vi "ROI entry-User ROI event-Analyse.vi"(8 "error in (no error)":errorcluster, 11 "Event Type":u32) -> (0 "error out":errorcluster, 2 "output cluster":T2 {"ROIs Info []"."Zoom" min=1.0 max=10.0 step=0.10000000149011612; "Last Image Display Event info"."Tool" items=["None", "Selection Tool", "Point Tool", "Line Tool", "Rectangle Tool", "Oval Tool", "Polygon Tool", "ClosedFreehandTool", "Annulus Tool", "Rotated Rectangle Tool", "Zoom Tool", "Pan Tool", "Polyline Tool", "Freehand Tool"]; "Last Image Display Event info"."Type" items=["No Event"=0, "Click Event"=1, "Draw Event"=2, "Size Event"=4, "Scroll Event"=5, "Double Click Event"=8]})   [LabVIEW 2013]
uses:
  Typedefs/ROI Entry screen VI interface 1.ctl
  Typedefs/Last Image Display Event info.ctl
  Typedefs/ROI spec.ctl
  Typedefs/ROI ID Enum.ctl
  Typedefs/ROI info cluster.ctl
  ROI Entry screen/Globals/gl_ROI Entry UI globals.vi
panel:
  out "ROI info cluster (native format)":T1
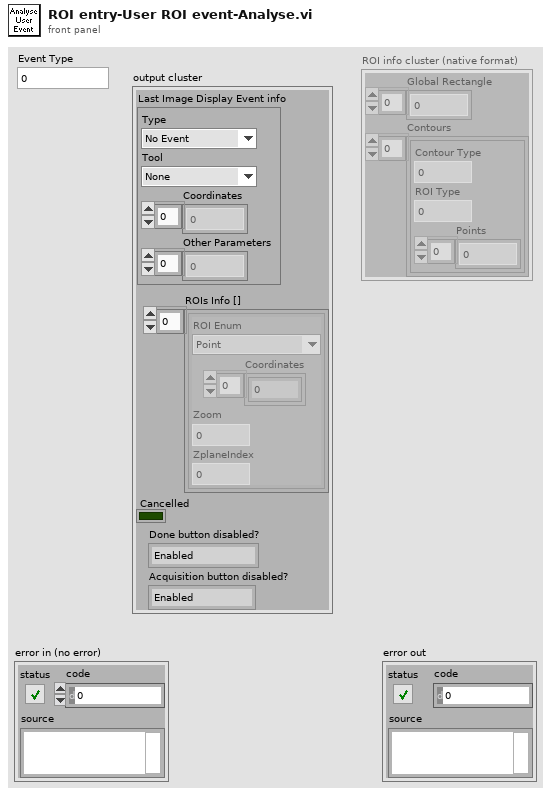
[diagram p1: front panel]
types:
  T1 = typedef "ROI info cluster.ctl" = cluster{"Global Rectangle":i32[], "Contours":cluster{"Contour Type":u32, "ROI Type":u32, "Points":i32[]}[]}
  T2 = typedef "ROI Entry screen VI interface 1.ctl" = cluster{"Last Image Display Event info":T3, "ROIs Info []":T4[], "Cancelled":bool, "Done button disabled?":enum8{"Enabled", "Disabled", "Disabled and Grayed Out"}, "Acquisition button disabled?":enum8{"Enabled", "Disabled", "Disabled and Grayed Out"}}
  T3 = typedef "Last Image Display Event info.ctl" = cluster{"Type":i32, "Tool":i32, "Coordinates":i32[], "Other Parameters":sgl[]}
  T4 = typedef "ROI spec.ctl" = cluster{"Coordinates":i32[], "Zoom":dbl, "ROI Enum":T5, "ZplaneIndex":i32}
  T5 = typedef "ROI ID Enum.ctl" = enum16{"Point", "MiniScan", "Comp. MiniScan", "Rectangle", "Comp. volume", "Arb. plane point"}
  T6 = typedef "ROI entry screen ctrl refs cluster.ctl" = cluster{"Done button":refnum<vi>, "Imaging button":refnum<vi>, "Acquisition button":refnum<vi>, "POI dwell time (us)":refnum<vi>, "Scan dwell time per pixel (us)":refnum<vi>, "# of planes":refnum<vi>, "Zoom":refnum<vi>, "Equal size":refnum<vi>, "Channel":refnum<vi>, "Image Display":refnum<vi>, "Z-Plane Selector":refnum<vi>, "Number of lines left":refnum<vi>, "Z-stack folder path":refnum<vi>, "POI Density":refnum<vi>, "Arb Plane Entry":refnum<vi>, "Whole plane":refnum<vi>, "Clear Last":refnum<vi>, "Clear All":refnum<vi>, "Trial Length (sec)":refnum<vi>, "Palette Type":refnum<vi>, "Intensity slider":refnum<vi>, "# POI":refnum<vi>, "Max Z Proj":refnum<vi>, "Zplane ind":refnum<vi>, "Wavelength (nm)":refnum<vi>, "Number of Trials":refnum<vi>, "Funct stim.trig.enable":refnum<vi>, "Funct stim.trig.delay (s)":refnum<vi>, "Line Mode":refnum<vi>, "Step size (µm)":refnum<vi>, "ROI move mode":refnum<vi>, "Cool-down time (s)":refnum<vi>, "Enable cool-down time":refnum<vi>, "Motor Z ind. (um)":refnum<vi>, "AOL Z ind. (um)":refnum<vi>}
  T7 = enum8{"Enabled", "Disabled", "Disabled and Grayed Out"}
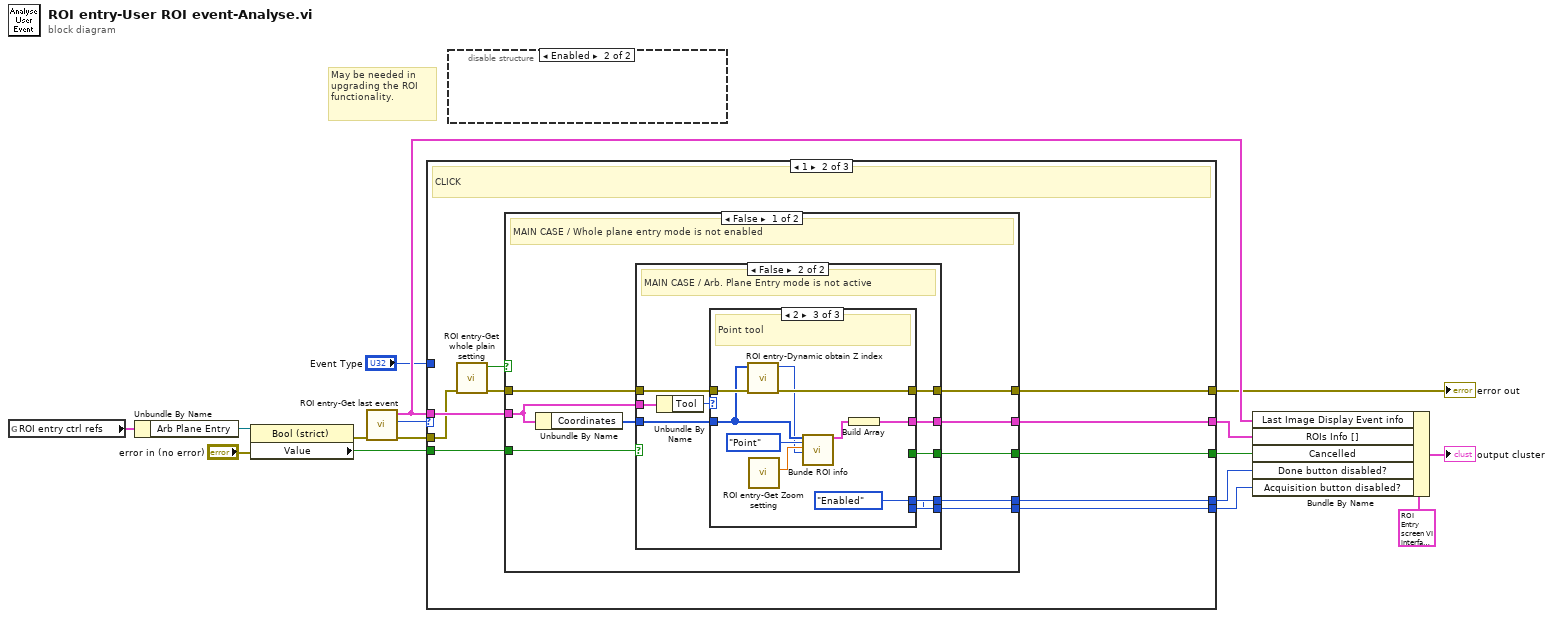
[diagram p0: block diagram]
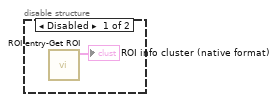
[diagram p2: hidden frame]
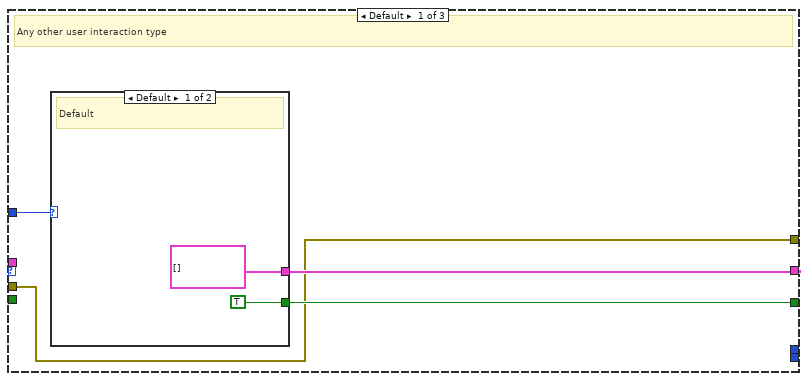
[diagram p3: hidden frame]
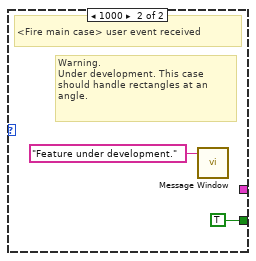
[diagram p4: hidden frame]
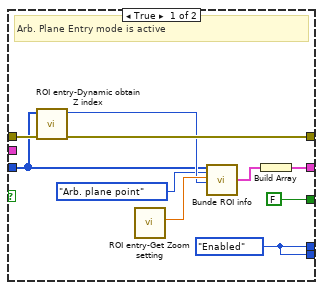
[diagram p5: hidden frame]
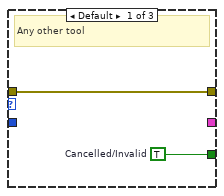
[diagram p6: hidden frame]
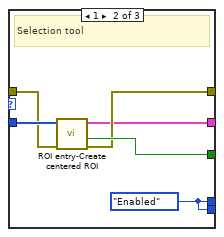
[diagram p7: hidden frame]
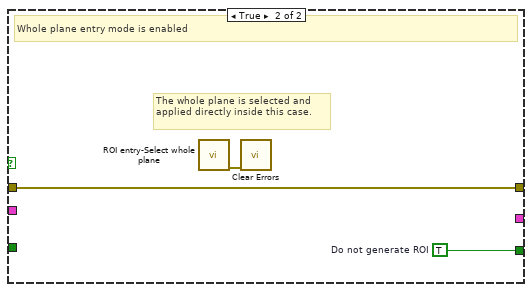
[diagram p8: hidden frame]
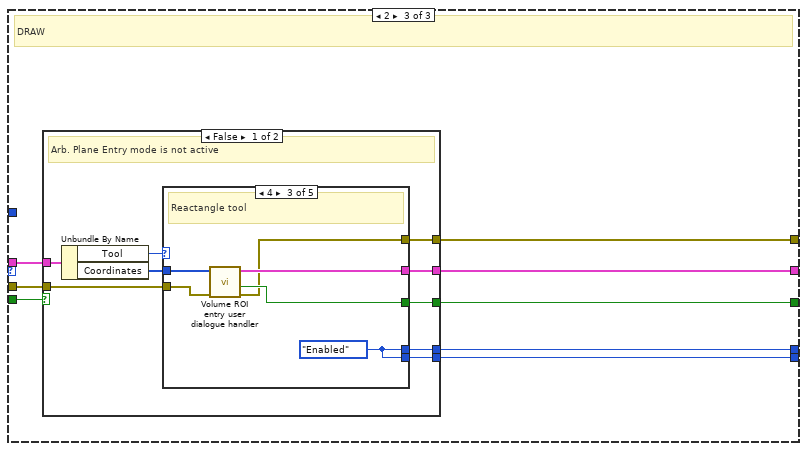
[diagram p9: hidden frame]
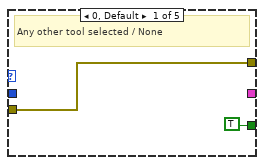
[diagram p10: hidden frame]
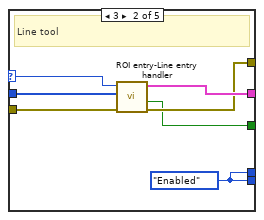
[diagram p11: hidden frame]
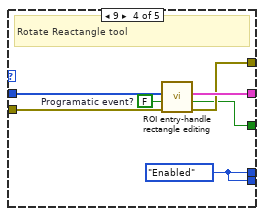
[diagram p12: hidden frame]
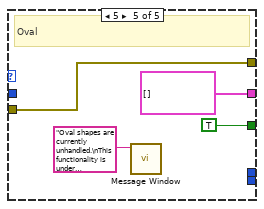
[diagram p13: hidden frame]
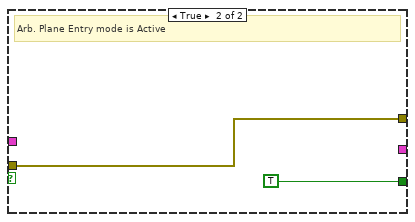
[diagram p14: hidden frame]
diagram:
  # "May be needed in upgrading the ROI functionality."
  n1 = global read "gl_ROI Entry UI globals.vi" "ROI entry ctrl refs"() -> (w15:T6)
  n2 = Unbundle By Name(w15) -> ("Arb Plane Entry"=w14:refnum<vi>)
  n3 = property class="Bool (strict)"(reference=w14, error in="error in (no error)") -> (error out=w4:errorcluster, "Value"=w16:bool)  [unwired: 1 out]
  n4 = call "ROI entry-Get last event.vi"("error in (no error)"=w4) -> ("error out"=w2:errorcluster, "Type"=w6:i32, "Last Image Display Event info"=w13:T3)  [unwired: 8 in]
  n5 = case shown="1" w6 {
    tunnel: [w19 w25 w90] -> w7
    tunnel: [w18 w34 w89] -> w11
    tunnel: [_ w33 w88] -> w8
    tunnel: [_ w32 w87] -> w9
    tunnel: "Event Type" -> [w20 _ _]
    tunnel: w16 -> [_ w31 w86]
    tunnel: w13 -> [_ w30 w85]
    tunnel: w2 -> [w17 w28 w83]
    tunnel: [w17 w26 w84] -> w1
    frame Default {
      # "Any other user interaction type"
      n6 = case shown="Default" w20 {
        tunnel: [T4[] [] ("ROIs Info []") _] -> w19
        tunnel: [TRUE TRUE ("Cancelled")] -> w18
        frame Default {
          # "Default"
        }
        frame 1000 {
          # "Warning.\nUnder development. This case should handle rectangles at an angle."
          # "<Fire main case> user event received"
          n7 = call "Message Window.vi"("Message string"="Feature under development." ("message")) -> ()  [unwired: 10 in, 1 out]
        }
      }
    }
    frame 1 {
      # "CLICK"
      n8 = call "ROI entry-Get whole plain setting.vi"("error in (no error)"=w28) -> ("error out"=w27:errorcluster, "\"Whole plain?\" value"=w29:bool)  [unwired: 9 in]
      n9 = case shown="False" w29 {
        tunnel: [w43 w82] -> w34
        tunnel: [w42 _] -> w33
        tunnel: [w41 _] -> w32
        tunnel: w31 -> [w40 _]
        tunnel: w30 -> [w38 _]
        tunnel: w27 -> [w35 w80]
        tunnel: [w36 w80] -> w26
        tunnel: [w37 _] -> w25
        frame False {
          # "MAIN CASE / Whole plane entry mode is not enabled"
          n10 = Unbundle By Name(w38) -> ("Coordinates"=w39:i32[])
          n11 = case shown="False" w40 {
            tunnel: w39 -> [w47 w62]
            tunnel: [FALSE ("Do not generate ROI") w61] -> w43
            tunnel: [w53 w60] -> w42
            tunnel: [w53 w59] -> w41
            tunnel: w38 -> [_ w58]
            tunnel: w35 -> [w51 w56]
            tunnel: [w50 w55] -> w36
            tunnel: [w46 w54] -> w37
            frame True {
              w53 = T7."Enabled" ("Disabled")
              # "Arb. Plane Entry mode is active"
              n12 = call "ROI entry-Dynamic obtain Z index.vi"("error in (no error)"=w51, "Coordinates"=w47) -> ("error out"=w50:errorcluster, "Z-plane selector (index)"=w48:i32)  [unwired: 8 in]
              n13 = call "ROI entry-Get Zoom setting.vi"() -> ("Zoom Value"=w49:dbl)  [unwired: 9 in, 2 out]
              n14 = call "Bunde ROI info.vi"("ROI Coordinates"=w47, "ROI Enum"=ROI_ID_Enum."Arb. plane point", "Zoom"=w49, "ZplaneIndex"=w48) -> ("ROI Info"=w45:T4)  [unwired: 15 in]
              n15 = Build Array(w45) -> (w46:T4[])
            }
            frame False {
              # "MAIN CASE / Arb. Plane Entry mode is not active"
              n16 = Unbundle By Name(w58) -> ("Tool"=w57:i32)
              n17 = case shown="2" w57 {
                tunnel: w62 -> [_ w69 w72]
                tunnel: [w64 w67 _] -> w61
                tunnel: [_ w70 w79] -> w60
                tunnel: [_ w70 w79] -> w59
                tunnel: w56 -> [w63 w68 w77]
                tunnel: [w63 w66 w78] -> w55
                tunnel: [_ w65 w75] -> w54
                frame Default {
                  w64 = TRUE  # Cancelled/Invalid
                  # "Any other tool"
                }
                frame 1 {
                  w70 = T7."Enabled" ("Disabled")
                  # "Selection tool"
                  n18 = call "ROI entry-Create centered ROI.vi"("error in (no error)"=w68, "Coordinates"=w69) -> ("error out"=w66:errorcluster, "Do not generate ROI"=w67:bool, "ROIs Info []"=w65:T4[])  [unwired: 7 in]
                }
                frame 2 {
                  w79 = T7."Enabled" ("Disabled")
                  # "Point tool"
                  n19 = call "ROI entry-Dynamic obtain Z index.vi"("error in (no error)"=w77, "Coordinates"=w72) -> ("error out"=w78:errorcluster, "Z-plane selector (index)"=w71:i32)  [unwired: 8 in]
                  n20 = call "ROI entry-Get Zoom setting.vi"() -> ("Zoom Value"=w76:dbl)  [unwired: 9 in, 2 out]
                  n21 = call "Bunde ROI info.vi"("ROI Coordinates"=w72, "ROI Enum"=ROI_ID_Enum."Point", "Zoom"=w76, "ZplaneIndex"=w71) -> ("ROI Info"=w74:T4)  [unwired: 15 in]
                  n22 = Build Array(w74) -> (w75:T4[])
                }
              }
            }
          }
        }
        frame True {
          w82 = TRUE  # Do not generate ROI
          # "The whole plane is selected and applied directly inside this case."
          # "Whole plane entry mode is enabled"
          n23 = call "ROI entry-Select whole plane.vi"() -> ("error IO"=w81:errorcluster)  [unwired: 11 in]
          n24 = call <vilib>:"Clear Errors.vi"("error in (no error)"=w81) -> ()  [unwired: 6 in, 1 out]
        }
      }
    }
    frame 2 {
      # "DRAW"
      n25 = case shown="False" w86 {
        tunnel: [w99 _] -> w90
        tunnel: [w98 TRUE ("Cancelled")] -> w89
        tunnel: [w97 _] -> w88
        tunnel: [w96 _] -> w87
        tunnel: w85 -> [w95 _]
        tunnel: [w91 w126] -> w84
        tunnel: w83 -> [w92 w126]
        frame False {
          # "Arb. Plane Entry mode is not active"
          n26 = Unbundle By Name(w95) -> ("Tool"=w94:i32, "Coordinates"=w93:i32[])
          n27 = case shown="4" w94 {
            selector: w94 -> [_ w105 _ _ _]
            tunnel: w93 -> [_ w106 w112 w119 _]
            tunnel: [_ w108 w114 w121 T4[] [] ("ROIs Info []")] -> w99
            tunnel: [TRUE w102 w110 w115 TRUE ("Cancelled")] -> w98
            tunnel: [_ w107 w113 w120 _] -> w97
            tunnel: [_ w107 w113 w120 _] -> w96
            tunnel: [w100 w104 w109 w116 w123] -> w91
            tunnel: w92 -> [w100 w103 w111 w117 w123]
            frame 0, Default {
              # "Any other tool selected / None"
            }
            frame 3 {
              w107 = T7."Enabled" ("Disabled")
              # "Line tool"
              n28 = call "ROI entry-Line entry handler.vi"("error in (no error)"=w103, "Coordinates"=w106, "Tool"=w105) -> ("error out"=w104:errorcluster, "Do not generate line ROI"=w102:bool, "Array"=w108:T4[])  [unwired: 6 in]
            }
            frame 4 {
              w113 = T7."Enabled" ("Disabled")
              # "Reactangle tool"
              n29 = call "Volume ROI entry user dialogue handler.vi"("error in (no error)"=w111, "New coordinates"=w112) -> ("error IO"=w109:errorcluster, "Cancelled"=w110:bool, "ROIs Info []"=w114:T4[])  [unwired: 7 in]
            }
            frame 9 {
              w118 = FALSE  # Programatic event?
              w120 = T7."Enabled" ("Disabled")
              # "Rotate Reactangle tool"
              n30 = call "ROI entry-handle rectangle editing.vi"("error in (no error)"=w117, "Programatic event?"=w118, "Coordinates"=w119) -> ("error IO"=w116:errorcluster, "Cancelled"=w115:bool, "ROIs Info []"=w121:T4[])  [unwired: 6 in]
            }
            frame 5 {
              # "Oval"
              n31 = call "Message Window.vi"("Message string"="Oval shapes are currently unhandled.\nThis functionality is under development." ("message")) -> ()  [unwired: 10 in, 1 out]
            }
          }
        }
        frame True {
          # "Arb. Plane Entry mode is Active"
        }
      }
    }
  }
  "error out" <- w1
  n32 = disable-structure shown="Enabled" {
    frame Disabled {
      n33 = call "ROI entry-Get ROI.vi"() -> ("ROI info cluster (native format)"=→"ROI info cluster (native format)":T1)  [unwired: 10 in, 1 out]
    }
    frame Enabled {
    }
  }
  n34 = Bundle By Name(cluster=T2 {"Last Image Display Event info"={"Type"=0, "Tool"=0, "Coordinates"=[], "Other Parameters"=[]}, "ROIs Info []"=[], "Cancelled"=FALSE, "Done button disabled?"=enum."Enabled", "Acquisition button disabled?"=enum."Enabled"} ("output cluster"), "Last Image Display Event info"=w13, "ROIs Info []"=w7, "Cancelled"=w11, "Done button disabled?"=w8, "Acquisition button disabled?"=w9) -> (→"output cluster":T2)
